vi "largeP_WRITE.vi"() -> ()   [LabVIEW 2009]
uses:
  <vilib>/Analysis/NI_AALBase.lvlib
panel:
  out "error out 2":errorcluster
  out "error out":errorcluster
  out "length":i32
  in  "dimension size":i32
  in  "sent":bool
  in  "stop":bool
  in  "Port":u16=64535
  in  "Machine":string="192.168.10.182"
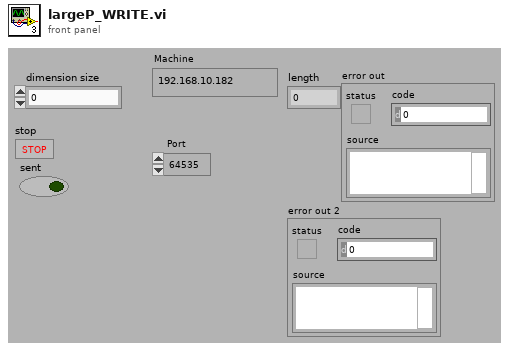
[diagram p1: front panel]
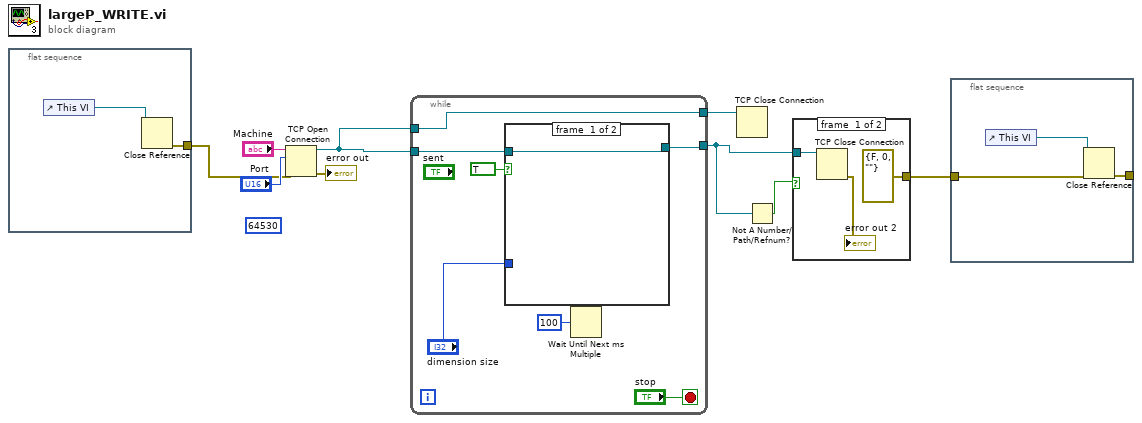
[diagram p0: block diagram]
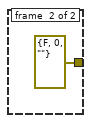
[diagram p2: hidden frame]
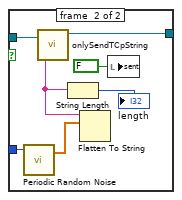
[diagram p3: hidden frame]
diagram:
  (unwired) u16 64530 ("local port (0)")
  n1 = flat-sequence {
    tunnel: [w10] -> w5
    frame #0 {
      n2 = control-ref of="This VI"() -> (w11:refnum<vi>)
      n3 = Close Reference(reference=w11) -> (error out=w10:errorcluster)  [unwired: 1 in]
    }
  }
  n4 = TCP Open Connection(address="Machine", remote port or service name="Port", error in (no error)=w5) -> (connection ID=w7:refnum<k5>, error out=→"error out":errorcluster)  [unwired: 2 out]
  n5 = while {
    tunnel: w7 -> [w18]
    tunnel: [w15] -> w4
    tunnel: w7 -> [w14]
    tunnel: [w14] -> w6
    stop <- "stop" stop-if-true
    n6 = case shown="True" TRUE {
      tunnel: w18 -> [w19 w26]
      tunnel: [w19 w24] -> w15
      tunnel: "dimension size" -> [_ w20]
      frame #0 {
      }
      frame #1 {
        n7 = call <vilib>:"Periodic Random Noise.vi"("samples"=w20) -> ("periodic random noise"=w21:dbl[])  [unwired: 2 in, 1 out]
        n8 = Flatten To String(anything=w21) -> (data string=w23:string)  [unwired: 3 in, 2 out]
        n9 = call "onlySendTCpString.vi"("imput string"=w23, "connection ID"=w26) -> ("connection ID out"=w24:refnum<k5>)  [unwired: 8 in, 1 out]
        n10 = String Length(string=w23) -> (length=→"length":i32)
        n11 = local write "sent"(FALSE ("sent")) -> ()
      }
    }
    n12 = Wait Until Next ms Multiple(millisecond multiple=u32 100) -> ()  [unwired: 1 out]
  }
  n13 = TCP Close Connection(connection ID=w6) -> ()  [unwired: 2 in, 2 out]
  n14 = Not A Number/Path/Refnum?(number/path/refnum=w4) -> (NaN/Path/Refnum?=w3:bool)
  n15 = case shown="False" w3 {
    tunnel: w4 -> [w29 _]
    tunnel: [errorcluster {"status"=FALSE, "code"=0, "source"=""} ("error out") errorcluster {"status"=FALSE, "code"=0, "source"=""} ("error out")] -> w2
    frame #0 {
      n16 = TCP Close Connection(connection ID=w29) -> (error out=→"error out 2":errorcluster)  [unwired: 2 in, 1 out]
    }
    frame #1 {
    }
  }
  n17 = flat-sequence {
    tunnel: [w32] -> _
    tunnel: w2 -> [w31]
    frame #0 {
      n18 = control-ref of="This VI"() -> (w33:refnum<vi>)
      n19 = Close Reference(reference=w33, error in (no error)=w31) -> (error out=w32:errorcluster)
    }
  }
